vi "On-Off Delay.vi"(6 "Off Delay":u32, 7 "OnDelay":u32, 11 "In":bool) -> (3 "Out":bool)   [LabVIEW 2021]
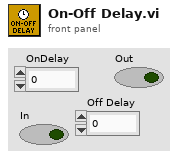
[diagram p1: front panel]
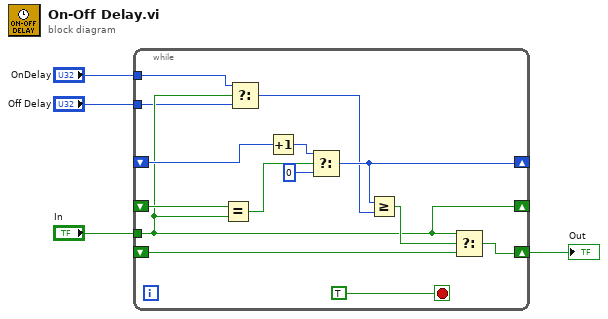
[diagram p0: block diagram]
diagram:
  n1 = while {
    tunnel: "In" -> [w8]
    shift-right: [w8] -> _
    shift-left: _ -> [w18]
    shift-right: [w12] -> _
    shift-left: _ -> [w14]
    shift-right: [w10] -> w3
    shift-left: _ -> [w9]
    tunnel: "OnDelay" -> [w6]
    tunnel: "Off Delay" -> [w7]
    stop <- TRUE stop-if-true
    n2 = Equal?(x=w18, y=w8) -> (x = y?=w15:bool)
    n3 = Select(t=w6, s=w8, f=w7) -> (s? t:f=w5:u32)
    n4 = Increment(x=w14) -> (x+1=w17:u32)
    n5 = Select(t=w17, s=w15, f=u32 0) -> (s? t:f=w12:u32)
    n6 = Greater Or Equal?(x=w12, y=w5) -> (x >= y?=w11:bool)
    n7 = Select(t=w8, s=w11, f=w9) -> (s? t:f=w10:bool)
  }
  "Out" <- w3
